vi "_Test_U8Array2Str.vi"(11 "Array":u8[](array[numeric])) -> (3 "data string":string)   [LabVIEW 2023]
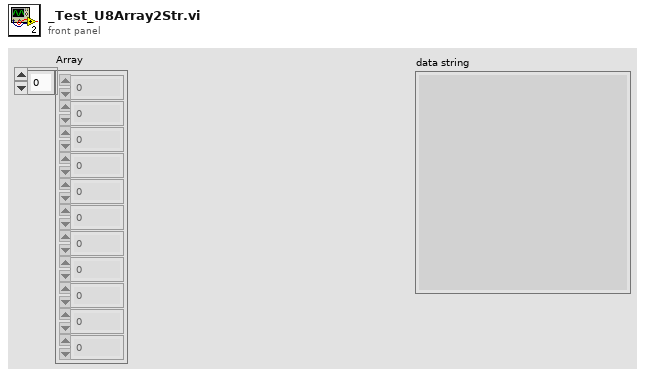
[diagram p1: front panel]
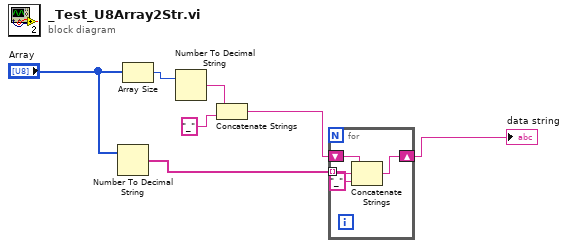
[diagram p0: block diagram]
diagram:
  n1 = Number To Decimal String(number="Array") -> (decimal integer string=w7:string[])  [unwired: 1 in]
  n2 = Array Size(array="Array") -> (size(s)=w4:i32)
  n3 = Number To Decimal String(number=w4) -> (decimal integer string=w3:string)  [unwired: 1 in]
  n4 = Concatenate Strings(w3, "_" ("string")) -> (w1:string)
  n5 = for {
    tunnel: w7 -> [w11] mode=indexing
    shift-right: [w10] -> w6
    shift-left: w1 -> [w9]
    n6 = Concatenate Strings(w9, w11, "_" ("string")) -> (w10:string)
  }
  "data string" <- w6
